vi "OTrig_h.vi"(8 "error in (no error)":errorcluster) -> (0 "error out":errorcluster)   [LabVIEW 2015, in "ESLSCDLL.lvlib"]
uses:
  ESLSCDLL.lvlib
  Globals.vi
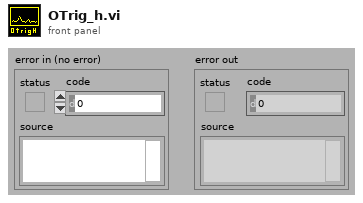
[diagram p1: front panel]
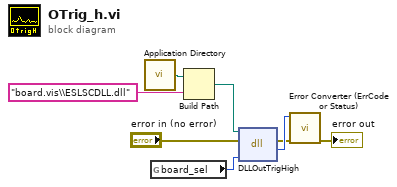
[diagram p0: block diagram]
diagram:
  n1 = call <vilib>:"Application Directory.vi"() -> ("Application Directory"=w4:path)
  n2 = global read "Globals.vi" "board_sel"() -> (w1:u32)
  n3 = Build Path(base path=w4, name or relative path="board.vis\\ESLSCDLL.dll") -> (appended path=w2:path)
  n4 = dll-call lib="C:/ENTW/PCIE/LV64/board.vis/ESLSCDLL.dll" fn="DLLOutTrigHigh"(path in=w2, error in="error in (no error)", "board_sel"=w1) -> (error out=w5:errorcluster, "es_status_codes"=w6:i32)  [unwired: 2 in, 1 out]
  n5 = call "Error Converter (ErrCode or Status).vi"("error in (no error)"=w5, "error code"=w6) -> ("error out"=→"error out":errorcluster)  [unwired: 9 in]
